vi "Write_parameter.vi"(8 "error in (no error)":errorcluster caption="entrée d'erreur (pas d'erreur)", 10 "Parameter":string, 11 "Class Instrument Firebase Altyor en entrée":refnum<class "Class Instrument Firebase Altyor.lvclass">) -> (0 "error out":errorcluster caption="sortie d'erreur", 3 "Class Instrument Firebase Altyor en sortie":refnum<class "Class Instrument Firebase Altyor.lvclass">)   [LabVIEW 2020, in "Library Instrument & Equipement.lvlib" / "Library Instruments.lvlib" / "Class Instrument Firebase Altyor.lvclass"]
uses:
  Class Instrument Firebase Altyor.lvclass
  Commun VI/TypeDef/Command firebase altyor/Parameter Firebase Altyor.ctl
  Commun VI/TypeDef/Bench Type.ctl
  Firebase/Source/Firebase Altyor/Firebase Altyor.lvclass
  JSON API/JSON Value/Set from JSON string.vi
  Instrument (Default)/Class Instrument (Default).lvclass
  JSON API/JSON Value/JSON Value.lvclass
  Class Instrument Firebase Altyor.lvclass/Class Instrument Firebase Altyor.ctl
  JSON API/Variant JSON/Variant JSON.lvlib
  JSON API/Get Polymorphic/JSON GetSet.lvlib
  Commun VI/Library Commun.lvlib
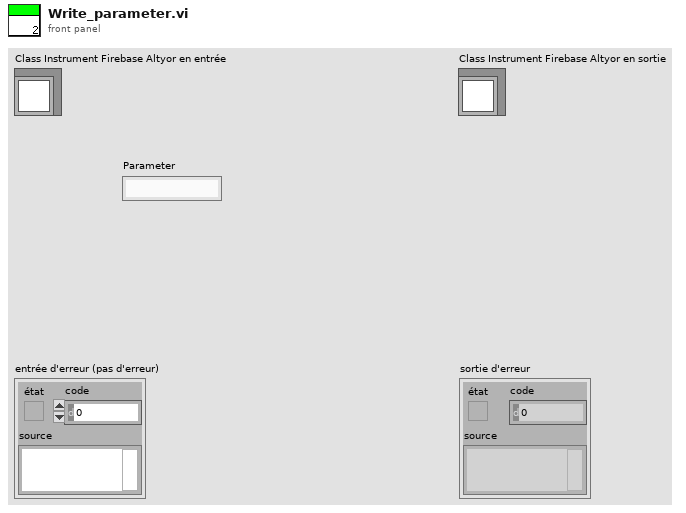
[diagram p1: front panel]
types:
  T1 = typedef "Library Commun.lvlib/Parameter Firebase Altyor.ctl" = cluster{"Name_BDD":string, "API_Key":string, "Nb_to_Read":string, "Value_to_find":string, "Field_Filter":string, "Field_Order":string, "Collection_to_find":string, "Name_Bench":string, "Bench Type":T2, "Type Data ":enum16{"Data Product", "Data Test"}, "Firebase Altyor":refnum<class "Firebase Altyor.lvclass">}
  T2 = typedef "Library Commun.lvlib/Bench Type.ctl" = enum16{"Bench PCBA", "Bench Camera", "Bench Assembly", "Bench PCBA P2193"}
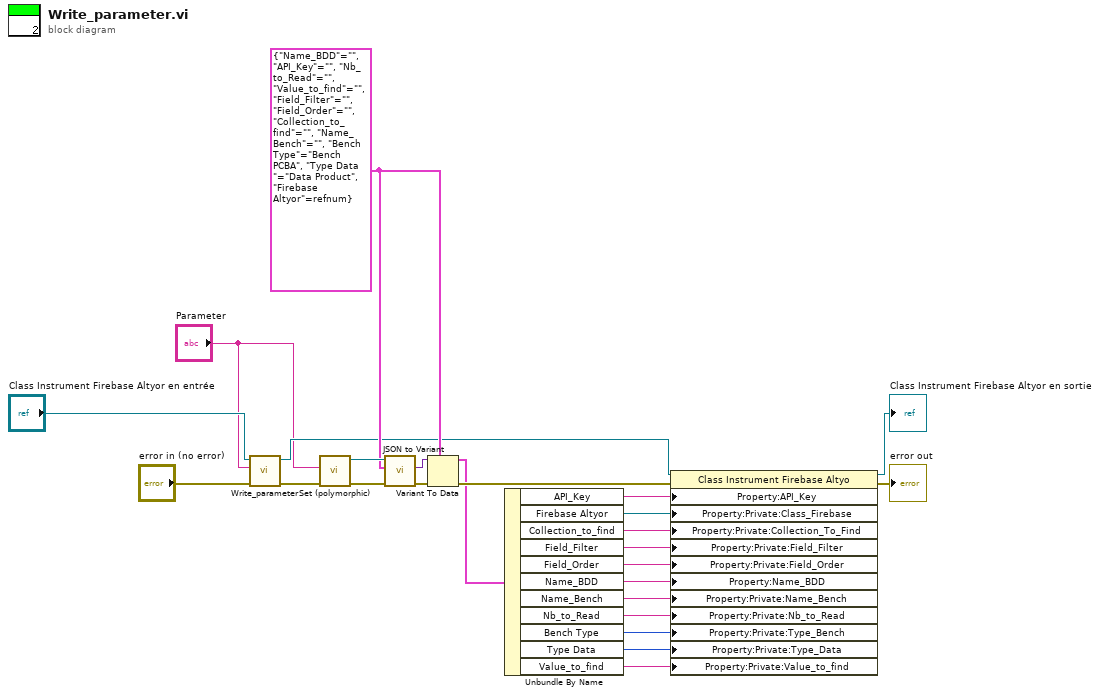
[diagram p0: block diagram]
diagram:
  w16 = T1 {"Name_BDD"="", "API_Key"="", "Nb_to_Read"="", "Value_to_find"="", "Field_Filter"="", "Field_Order"="", "Collection_to_find"="", "Name_Bench"="", "Bench Type"=enum."Bench PCBA", "Type Data "=enum."Data Product", "Firebase Altyor"=refnum} ("Parameter")
  n1 = call-parent "Write_parameter.vi"("error in (no error)"="error in (no error)", "Parameter"="Parameter", "Class Instrument (Default) en entrée"="Class Instrument Firebase Altyor en entrée") -> ("error out"=w4:errorcluster, "Class Instrument (Default) en sortie"=w2:refnum<class "Class Instrument Firebase Altyor.lvclass">)  [unwired: 7 in]
  n2 = call-poly "Set (polymorphic).vi"("error in (no error)"=w4, "JSON stream"="Parameter") -> ("error out"=w23:errorcluster, "JSON Value out"=w25:refnum<class "JSON Value.lvclass">)  [unwired: 7 in, 1 out]
  n3 = call "JSON to Variant.vi"("error in (no error)"=w23, "Variant (Data Type)"=w16, "JSON Value"=w25) -> ("error out"=w24:errorcluster, "Variant out"=w22:variant)  [unwired: 7 in]
  n4 = Variant To Data(error in=w24, type=w16, Variant=w22) -> (data=w17:T1, error out=w19:errorcluster)
  n5 = Unbundle By Name(w17) -> ("API_Key"=w15:string, "Firebase Altyor"=w14:refnum<class "Firebase Altyor.lvclass">, "Collection_to_find"=w13:string, "Field_Filter"=w12:string, "Field_Order"=w11:string, "Name_BDD"=w10:string, "Name_Bench"=w9:string, "Nb_to_Read"=w8:string, "Bench Type"=w7:T2, "Type Data"=w6:enum16{"Data Product", "Data Test"}, "Value_to_find"=w5:string)
  n6 = property class="Class Instrument Firebase Altyo"(reference=w2, error in=w19, "Property:API_Key"=w15, "Property:Private:Class_Firebase"=w14, "Property:Private:Collection_To_Find"=w13, "Property:Private:Field_Filter"=w12, "Property:Private:Field_Order"=w11, "Property:Name_BDD"=w10, "Property:Private:Name_Bench"=w9, "Property:Private:Nb_to_Read"=w8, "Property:Private:Type_Bench"=w7, "Property:Private:Type_Data"=w6, "Property:Private:Value_to_find"=w5) -> (reference out=→"Class Instrument Firebase Altyor en sortie":refnum<class "Class Instrument Firebase Altyor.lvclass">, error out=→"error out":errorcluster)
